vi "Construct Pipes.vi"() -> ()   [LabVIEW 2015]
panel:
  out "Syringe":bool
  out "Syringe pipe 3":bool
  out "Syringe pipe 2":bool
  out "Syringe pipe 1":bool
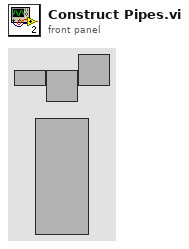
[diagram p1: front panel]
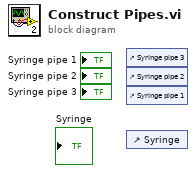
[diagram p0: block diagram]
diagram:
  n1 = control-ref of="Syringe pipe 3"() -> ()  [unwired: 1 out]
  n2 = control-ref of="Syringe pipe 2"() -> ()  [unwired: 1 out]
  n3 = control-ref of="Syringe pipe 1"() -> ()  [unwired: 1 out]
  n4 = control-ref of="Syringe"() -> ()  [unwired: 1 out]
